vi "kalmanf.vi"(0 "u":T1, 1 "A":T1, 2 "B":T1, 3 "C":T1, 5 "y":T1, 9 "Q":T1, 11 "R":T1, 12 "xhat0":T1, 13 "P0":T1) -> (4 "xhat":T1)   [LabVIEW 2018]
uses:
  <vilib>/Analysis/Matrix/Datatypes/RealMatrix.ctl
  <vilib>/Analysis/baseanly.llb/Real A x B.vi
  <vilib>/Analysis/7linalg.llb/Real Transpose Matrix.vi
  <vilib>/Analysis/Matrix/Numeric/Add/Add - RM,RM.vi
  <vilib>/Analysis/Matrix/Numeric/Subtract/Subtract - RM,RM.vi
  <vilib>/Analysis/baseanly.llb/Real Inverse Matrix.vi
  <vilib>/Analysis/NI_AALBase.lvlib
  <vilib>/Analysis/NI_AALPro.lvlib
  <vilib>/Analysis/Matrix/NI_Matrix.lvlib
panel:
  # "Initial values:\n========="
  # "x(k) = Ax(k-1)+Bu(k-1)+v\ny(k) = Cx(k)+w\n\nv = N(0, Q^2)\nw = N(0, R^2)\n\nxhat : estimated system states"
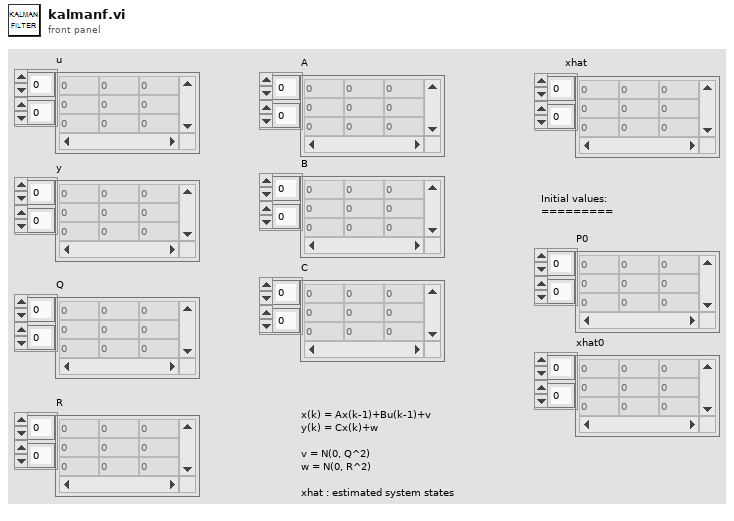
[diagram p1: front panel]
types:
  T1 = typedef "NI_Matrix.lvlib/RealMatrix.ctl" = dbl[][]
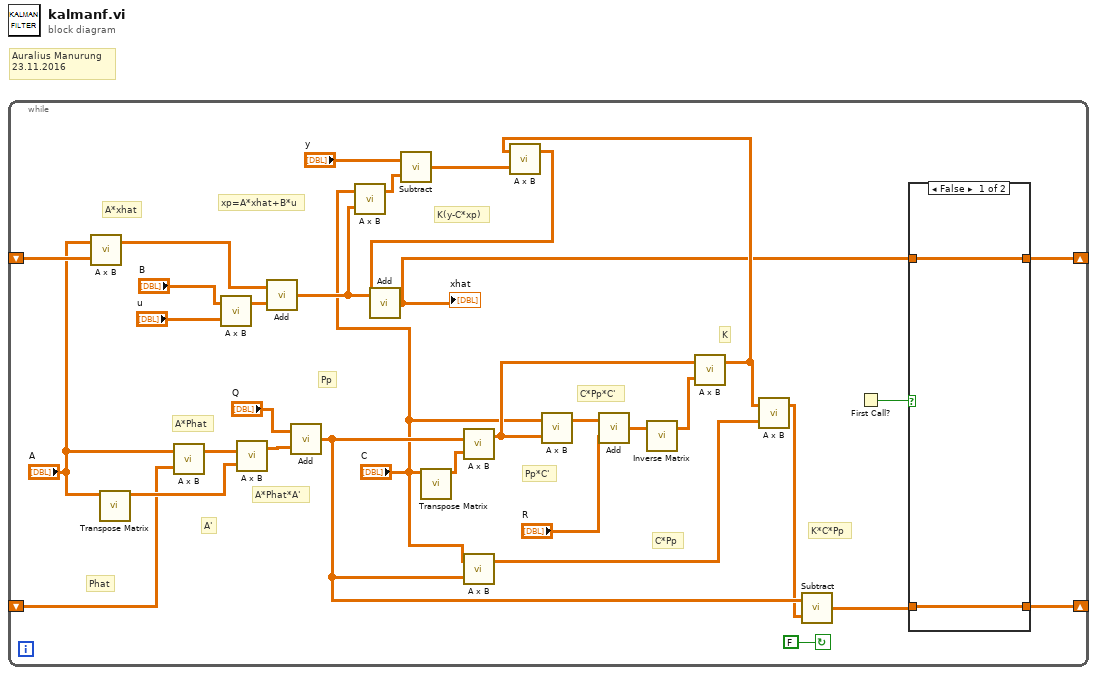
[diagram p0: block diagram]
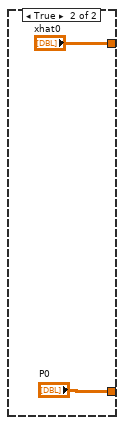
[diagram p2: hidden frame]
diagram:
  # "Auralius Manurung\n23.11.2016"
  n1 = while {
    shift-right: [w3] -> _
    shift-left: _ -> [w19]
    shift-right: [w5] -> _
    shift-left: _ -> [w15]
    stop <- FALSE continue-if-true
    # "K(y-C*xp)"
    # "xp=A*xhat+B*u"
    # "A*xhat"
    # "K*C*Pp"
    # "A*Phat*A'"
    # "Phat"
    # "A*Phat"
    # "K"
    # "C*Pp"
    # "Pp*C'"
    # "C*Pp*C'"
    # "A'"
    # "Pp"
    n2 = call-poly <vilib>:"A x B.vi"("B"=w15, "A"="A") -> ("A x B"=w13:T1)  [unwired: 1 out]
    n3 = call-poly <vilib>:"Transpose Matrix.vi"("Input Matrix"="A") -> ("Matrix Transpose"=w31:T1)  [unwired: 9 in, 1 out]
    n4 = call-poly <vilib>:"A x B.vi"("B"=w19, "A"="A") -> ("A x B"=w30:T1)  [unwired: 1 out]
    n5 = call-poly <vilib>:"A x B.vi"("B"="u", "A"="B") -> ("A x B"=w16:T1)  [unwired: 1 out]
    n6 = call-poly <vilib>:"A x B.vi"("B"=w31, "A"=w30) -> ("A x B"=w33:T1)  [unwired: 1 out]
    n7 = call-poly <vilib>:"Add.vi"("Real Matrix B"=w16, "Real Matrix A"=w13) -> ("A + B"=w12:T1)
    n8 = call-poly <vilib>:"Add.vi"("Real Matrix B"=w33, "Real Matrix A"="Q") -> ("A + B"=w23:T1)
    n9 = call-poly <vilib>:"A x B.vi"("B"=w12, "A"="C") -> ("A x B"=w11:T1)  [unwired: 1 out]
    n10 = call-poly <vilib>:"Subtract.vi"("Real Matrix B"=w11, "Real Matrix A"="y") -> ("A - B"=w9:T1)
    n11 = call-poly <vilib>:"Transpose Matrix.vi"("Input Matrix"="C") -> ("Matrix Transpose"=w29:T1)  [unwired: 9 in, 1 out]
    n12 = call-poly <vilib>:"A x B.vi"("B"=w29, "A"=w23) -> ("A x B"=w24:T1)  [unwired: 1 out]
    n13 = call-poly <vilib>:"A x B.vi"("B"=w23, "A"="C") -> ("A x B"=w22:T1)  [unwired: 1 out]
    n14 = call-poly <vilib>:"A x B.vi"("B"=w24, "A"="C") -> ("A x B"=w28:T1)  [unwired: 1 out]
    n15 = call-poly <vilib>:"Add.vi"("Real Matrix B"="R", "Real Matrix A"=w28) -> ("A + B"=w26:T1)
    n16 = call-poly <vilib>:"Inverse Matrix.vi"("Input Matrix"=w26) -> ("Inverse Matrix"=w25:T1)  [unwired: 1 in, 1 out]
    n17 = call-poly <vilib>:"A x B.vi"("B"=w25, "A"=w24) -> ("A x B"=w8:T1)  [unwired: 1 out]
    n18 = call-poly <vilib>:"A x B.vi"("B"=w9, "A"=w8) -> ("A x B"=w7:T1)  [unwired: 1 out]
    n19 = call-poly <vilib>:"Add.vi"("Real Matrix B"=w7, "Real Matrix A"=w12) -> ("A + B"=w4:T1)
    "xhat" <- w4
    n20 = call-poly <vilib>:"A x B.vi"("B"=w22, "A"=w8) -> ("A x B"=w21:T1)  [unwired: 1 out]
    n21 = call-poly <vilib>:"Subtract.vi"("Real Matrix B"=w21, "Real Matrix A"=w23) -> ("A - B"=w2:T1)
    n22 = First Call?() -> (First Call?: T/F=w6:bool)
    n23 = case shown="False" w6 {
      tunnel: [w35 "xhat0"] -> w5
      tunnel: w4 -> [w35 _]
      tunnel: [w34 "P0"] -> w3
      tunnel: w2 -> [w34 _]
      frame False {
      }
      frame True {
      }
    }
  }
